vi "Push Backup to DB.vi"(7 "Backup lines at a time":i32=1000, 9 "timestamp string":string, 10 "Path to backup file":path, 11 "Data.PG in":refnum<class "Data.PG.lvclass">) -> ()   [LabVIEW 2020, in "Data.PG.lvclass"]
uses:
  Data.PG.lvclass
  Data.PG.lvclass/Data.PG.ctl
  <vilib>/JDP Science/PostgreSQL Library/Result/PQ Result.lvclass/PQ Result.ctl
  <vilib>/JDP Science/PostgreSQL Library/Connection/Execute Command (No results).vi
  <vilib>/JDP Science/PostgreSQL Library/Result/Clear.vi
  <vilib>/JDP Science/PostgreSQL Library/Connection/Execute Command (Result).vi
  <vilib>/JDP Science/PostgreSQL Library/Connection/Execute (Return first result with rows).vi
  <vilib>/JDP Science/PostgreSQL Library/Connection/Single Command with parameters.vi
  <vilib>/JDP Science/PostgreSQL Library/Connection/PQ Connection.lvclass
panel:
  out "Success?":bool
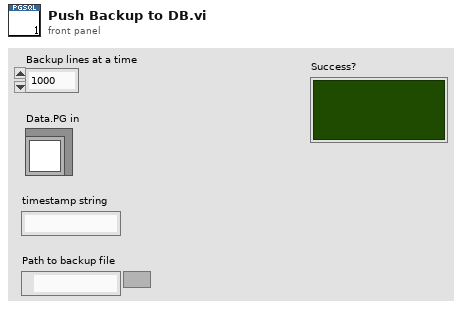
[diagram p1: front panel]
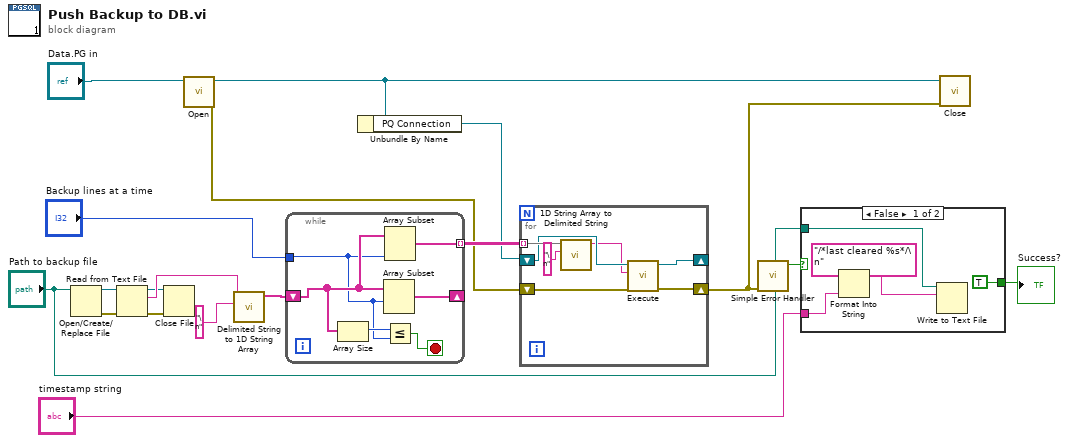
[diagram p0: block diagram]
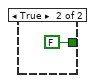
[diagram p2: hidden frame]
diagram:
  n1 = Open/Create/Replace File(file path (use dialog)="Path to backup file") -> (refnum out=w17:refnum<file>, error out=w18:errorcluster)  [unwired: 5 in, 1 out]
  n2 = Read from Text File(file (use dialog)=w17, error in=w18) -> (refnum out=w3:refnum<file>, text=w16:string, error out=w2:errorcluster)  [unwired: 2 in, 1 out]
  n3 = Close File(refnum=w3, error in=w2) -> ()  [unwired: 2 out]
  n4 = call-dynamic "Open.vi"("Data.PG in"="Data.PG in") -> ("error out"=w10:errorcluster, "Data.PG out"=w9:refnum<class "Data.PG.lvclass">)  [unwired: 9 in]
  n5 = call <vilib>:"Delimited String to 1D String Array.vi"("delimiter"="\n", "delimited string"=w16) -> ("string array"=w14:string[])  [unwired: 9 in]
  n6 = while {
    shift-right: [w24] -> _
    shift-left: w14 -> [w23]
    tunnel: [w20] -> w12 mode=indexing
    tunnel: "Backup lines at a time" -> [w19]
    stop <- w21 stop-if-true
    n7 = Array Size(array=w23) -> (size(s)=w22:i32)
    n8 = Array Subset(array=w23, index=w19) -> (w24:string[])  [unwired: 1 in]
    n9 = Array Subset(array=w23, length=w19) -> (w20:string[])  [unwired: 1 in]
    n10 = Less Or Equal?(x=w22, y=w19) -> (x <= y?=w21:bool)
  }
  n11 = Unbundle By Name(w9) -> ("PQ Connection"=w8:refnum<class "PQ Connection.lvclass">)
  n12 = for {
    tunnel: w12 -> [w30] mode=indexing
    shift-right: [w29] -> w7
    shift-left: w10 -> [w28]
    shift-right: [w27] -> _
    shift-left: w8 -> [w26]
    n13 = call <vilib>:"1D String Array to Delimited String.vi"("delimiter"="\n", "string array"=w30) -> ("delimited string"=w25:string)  [unwired: 9 in]
    n14 = call-poly <vilib>:"Execute.vi"("error in (no error)"=w28, "SQL"=w25, "PQ Connection in"=w26) -> ("error out"=w29:errorcluster, "PQ Connection out"=w27:refnum<class "PQ Connection.lvclass">)  [unwired: 7 in]
  }
  n15 = call <vilib>:"Simple Error Handler.vi"("error in (no error)"=w7) -> ("error?"=w6:bool)  [unwired: 4 in, 4 out]
  n16 = case shown="False" w6 {
    tunnel: "Path to backup file" -> [w34 _]
    tunnel: "timestamp string" -> [w35 _]
    tunnel: [TRUE FALSE] -> w1
    frame False {
      n17 = Format Into String(format string="/*last cleared %s*/\n", w35) -> (resulting string=w33:string)  [unwired: 2 in, 1 out]
      n18 = Write to Text File(file (use dialog)=w34, text=w33) -> ()  [unwired: 2 in, 3 out]
    }
    frame True {
    }
  }
  "Success?" <- w1
  n19 = call-dynamic "Close.vi"("error in (no error)"=w7, "Data.PG in"=w9) -> ()  [unwired: 8 in, 2 out]
